vi "Digest Error.vi"(8 "error in (no error)":errorcluster, 10 "Error Infor":T1 {"Time Stamp" format="%<%x %.3X>T"}, 11 "Local Error Manager in":refnum<class "Local Error Manager.lvclass">) -> (0 "error out":errorcluster, 3 "Local Error Manager out":refnum<class "Local Error Manager.lvclass">)   [LabVIEW 2026, in "TALOS.lvlib" / "Error Manager.lvlib" / "Local Error Manager.lvclass"]
uses:
  Local Error Manager.lvclass
  C:/LabVIEW Code/TALOS/talos/Internal uServices/System uServices/Error Manager/Error Manager.lvclass
  C:/LabVIEW Code/TALOS/talos/Father of all uServices/Father of all uServices/Father of all uServices.lvclass
  Error Info.ctl
  Error Manager.lvclass/Error Manager.ctl
  <vilib>/Utility/error.llb/DialogType.ctl
  Guardian/Guardian Messages/Message to uService Msg/Message to uService Msg.lvclass/Message to uService Msg.ctl
  Ancestor/Ancestor/Ancestor.lvclass/Ancestor.ctl
  Write Distributed Error Manager Started flag.vi
  Read Distributed Error Manager Started flag.vi
  Read Distributed flag.vi
  FGV/Error Memory/Get All Errors Arrays.vi
  Guardian/Guardian Messages/Message to uService Msg/Send Message to uService.vi
  Support VIs/Generate Error.vi
  FGV/Error Memory/Error Memory Core.vi
  FGV/Error Memory/Get Error Description.vi
  Support VIs/Get PC name.vi
  Ancestor/Ancestor/Read ID.vi
  Support VIs/Get Class Name.vi
  Support VIs/Circus Root Path.vi
  FGV/Error Memory/Error Crt Lvl checker.vi
  FGV/Error Memory/Error Memory Core.vi/40c8088d-b597-4017-91af-faa98e00292e.vi
  FGV/Error Memory/Error Memory Core.vi/d4a3ab98-063c-4e44-b43d-fbdcfe6c2be2.vi
  <vilib>/AdvancedString/Delimited String to 1D String Array.vi
  <vilib>/AdvancedString/Delimited String to 1D String Array (string).vi
  Father of all uServices/Father of all uServices/Father of all uServices.lvclass
  C:/LabVIEW Code/TALOS/builds/Actor Framework PPL/Actor Framework.lvlibp/1abvi3w/vi.lib/ActorFramework/Actor/Actor.lvclass
  Support VIs/Is in Packed Library.vi
  Support VIs/TALOS Root path.vi
  Support VIs/Read CSV worksheet.vi
  Support VIs/Global Memory.vi
  Support VIs/Global Constants.vi
  <vilib>/Utility/error.llb/General Error Handler.vi
  builds/Actor Framework PPL/Actor Framework.lvlibp/1abvi3w/vi.lib/ActorFramework/Actor/Read Caller Enqueuer.vi
  builds/Actor Framework PPL/Actor Framework.lvlibp/1abvi3w/vi.lib/ActorFramework/Message Enqueuer/Enqueue.vi
  <vilib>/Utility/LVClass/Get LV Class Name.vi
  Support VIs/Error Log.vi
  <vilib>/Comparison/Equal/Equal Functor/Equal Functor.lvclass
  Guardian/Guardian Messages/Message to uService Msg/Message to uService Msg.lvclass
  Ancestor/Ancestor/Ancestor.lvclass
  Classes/Error Filter/Error Filter.lvclass
  TALOS.lvlib
  Error Manager.lvclass
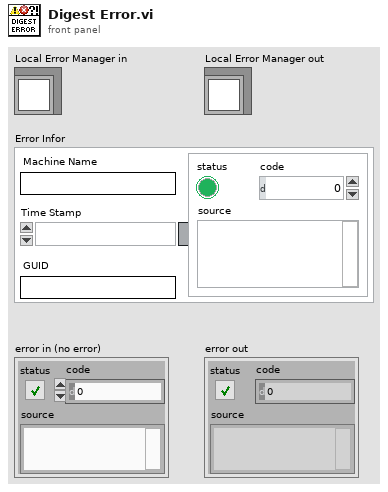
[diagram p1: front panel]
types:
  T1 = typedef "TALOS.lvlib/Error Manager.lvlib/Error Manager.lvclass/Error Info.ctl" = cluster{"error out":errorcluster, "Time Stamp":timestamp, "Machine Name":string, "GUID":string}
  T2 = typedef "DialogType.ctl" = u16
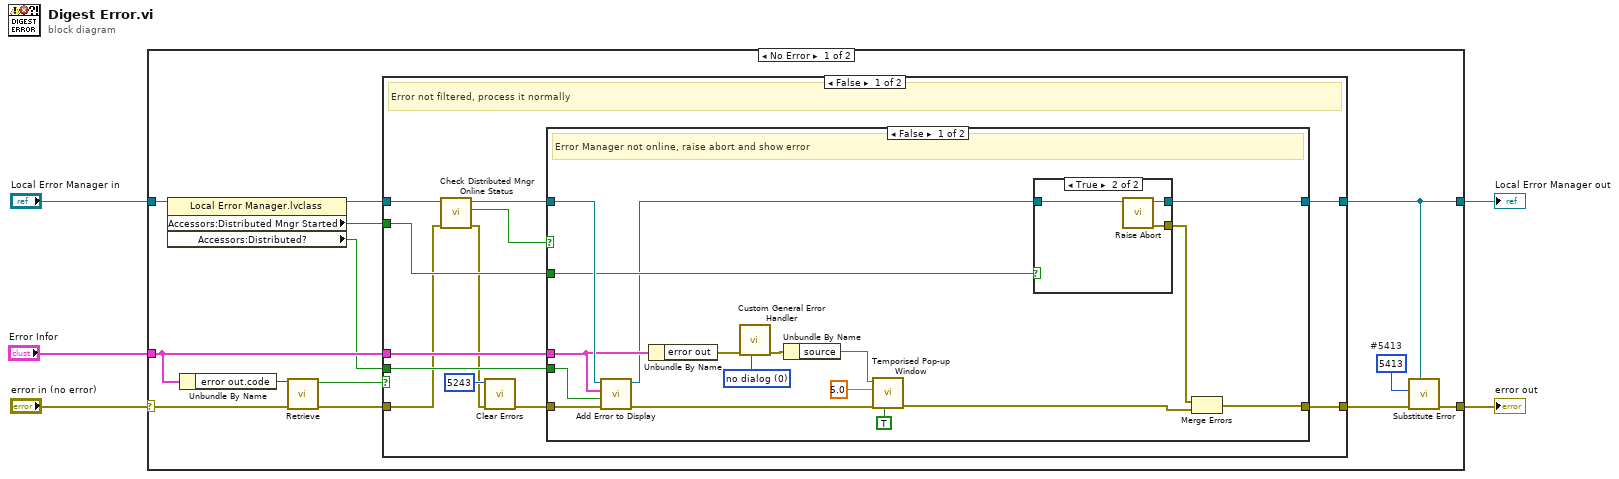
[diagram p0: block diagram]
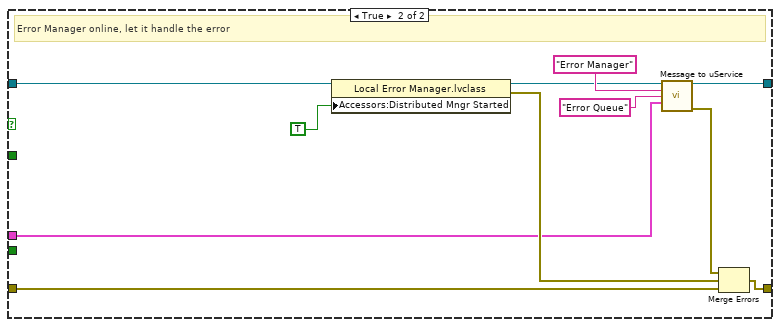
[diagram p3: hidden frame]
diagram:
  n1 = case shown="No Error" "error in (no error)" {
    selector: "error in (no error)" -> [w13 w65]
    tunnel: "Error Infor" -> [w16 _]
    tunnel: "Local Error Manager in" -> [w15 w66]
    tunnel: [w7 w65] -> w3
    tunnel: [w6 w66] -> w4
    frame No Error {
      w9 = 5413  # #5413
      n2 = property class="Local Error Manager.lvclass"(reference=w15) -> (reference out=w12:refnum<class "Local Error Manager.lvclass">, "Accessors:Distributed Mngr Started"=w11:bool, "Accessors:Distributed?"=w10:bool)  [unwired: 1 in, 1 out]
      n3 = Unbundle By Name(w16) -> ("error out.code"=w14:i32)
      n4 = call "Retrieve.vi"("error in (no error)"=w13, "Error Code"=w14) -> ("error out"=w18:errorcluster, "Filter?"=w17:bool)  [unwired: 8 in]
      n5 = case shown="False" w17 {
        tunnel: w12 -> [w23 w64]
        tunnel: [w25 w64] -> w6
        tunnel: [w30 w63] -> w8
        tunnel: w18 -> [w19 w63]
        tunnel: w16 -> [w29 _]
        tunnel: w11 -> [w26 _]
        tunnel: w10 -> [w24 _]
        frame False {
          # "Error not filtered, process it normally"
          n6 = call "Check Distributed Mngr Online Status.vi"("error in (no error)"=w19, "Local Error Manager in"=w23) -> ("error out"=w20:errorcluster, "uService online"=w21:bool, "Local Error Manager out"=w22:refnum<class "Local Error Manager.lvclass">)  [unwired: 7 in]
          n7 = call <vilib>:"Clear Errors.vi"("error in (no error)"=w20, "specific error code to clear (0: all)"=5243) -> ("error out"=w28:errorcluster)  [unwired: 4 in, 1 out]
          n8 = case shown="False" w21 {
            tunnel: [w35 w58] -> w25
            tunnel: [w33 w62] -> w30
            tunnel: w28 -> [w46 w57]
            tunnel: w22 -> [w45 w52]
            tunnel: w29 -> [w42 w54]
            tunnel: w26 -> [w37 _]
            tunnel: w24 -> [w31 _]
            frame False {
              w44 = T2 0 items=["no dialog", "OK message", "continue or stop message", "OK message + warnings", "continue/stop + warnings"] ("type of dialog (OK msg:1)")
              # "Error Manager not online, raise abort and show error"
              n9 = call "Add Error to Display.vi"("error in (no error)"=w46, "Update Listbox"=w31, "error to display"=w42, "Error Manager in"=w45) -> ("error out"=w43:errorcluster, "Error Manager out"=w36:refnum<class "Local Error Manager.lvclass">)  [unwired: 6 in]
              n10 = Unbundle By Name(w42) -> ("error out"=w41:errorcluster)
              n11 = call "Custom General Error Handler.vi"("type of dialog (OK msg:1)"=w44, "error in (no error)"=w41) -> ("error out"=w39:errorcluster)  [unwired: 9 in]
              n12 = Unbundle By Name(w39) -> ("source"=w40:string)
              n13 = call "Temporised Pop-up Window.vi"("error window"=TRUE, "error in (no error)"=w43, "Timeout"=5.0, "Text"=w40) -> ("error out"=w32:errorcluster)  [unwired: 7 in]
              n14 = case shown="True" w37 {
                tunnel: w36 -> [w48 w51]
                tunnel: [w48 w50] -> w35
                tunnel: [_ w49] -> w34
                frame False {
                }
                frame True {
                  n15 = call "Raise Abort.vi"("Father of all uServices in"=w51) -> ("error out"=w49:errorcluster, "Father of all uServices out"=w50:refnum<class "Local Error Manager.lvclass">)  [unwired: 9 in]
                }
              }
              n16 = Merge Errors(w34, w32) -> (w33:errorcluster)
            }
            frame True {
              # "Error Manager online, let it handle the error"
              n17 = property class="Local Error Manager.lvclass"(reference=w52, "Accessors:Distributed Mngr Started"=TRUE ("Global Mgr Started")) -> (reference out=w59:refnum<class "Local Error Manager.lvclass">, error out=w56:errorcluster)  [unwired: 1 in]
              n18 = call "Message to uService.vi"("Father of all uServices in"=w59, "uService ID"="Error Manager", "Message"="Error Queue", "Data"=w54) -> ("Father of all uServices out"=w58:refnum<class "Local Error Manager.lvclass">, "error out"=w55:errorcluster)  [unwired: 10 in]
              n19 = Merge Errors(w55, w56, w57) -> (w62:errorcluster)
            }
          }
        }
        frame True {
          # "Error filtered, skip it"
        }
      }
      n20 = call "Substitute Error.vi"("LabVIEW Object"=w6, "error in (no error)"=w8, "Error Code"=w9) -> ("error out"=w7:errorcluster)  [unwired: 8 in]
    }
    frame Error {
    }
  }
  "Local Error Manager out" <- w4
  "error out" <- w3
